vi "Apply.vi"(8 "error in (no error)":errorcluster, 11 "PXIe-5172:Fetch Waveforms CFG in":refnum<class "Voltmeter CFG.lvclass">=refnum) -> (0 "error out":errorcluster, 3 "PXIe-5172:Fetch Waveforms CFG out":refnum<class "Voltmeter CFG.lvclass">)   [LabVIEW 2023, in "PXIe-5172.lvlib" / "Fetch Waveforms CFG.lvclass"]
uses:
  Fetch Waveforms CFG.lvclass
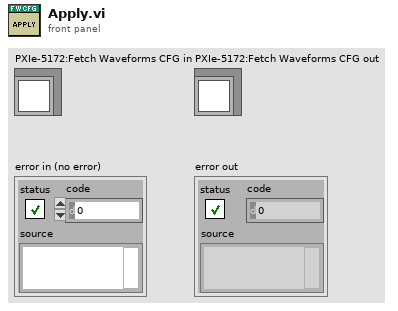
[diagram p1: front panel]
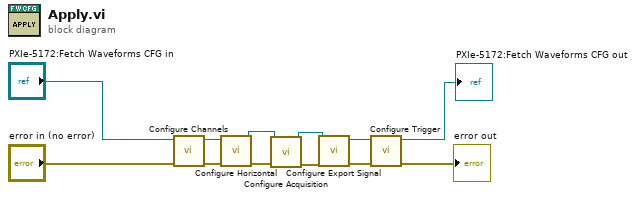
[diagram p0: block diagram]
diagram:
  n1 = call-dynamic "Configure Channels.vi"("error in"="error in (no error)", "Scope PXI CFG in"="PXIe-5172:Fetch Waveforms CFG in") -> ("error out"=w11:errorcluster, "Scope PXI CFG out"=w12:refnum<class "Voltmeter CFG.lvclass">)  [unwired: 8 in]
  n2 = call-dynamic "Configure Horizontal.vi"("error in"=w11, "Scope PXI CFG in"=w12) -> ("error out"=w7:errorcluster, "Scope PXI CFG out"=w8:refnum<class "Voltmeter CFG.lvclass">)  [unwired: 8 in]
  n3 = call-dynamic "Configure Acquisition.vi"("error in"=w7, "Scope PXI CFG in"=w8) -> ("error out"=w5:errorcluster, "Scope PXI CFG out"=w6:refnum<class "Voltmeter CFG.lvclass">)  [unwired: 8 in]
  n4 = call-dynamic "Configure Export Signal.vi"("error in"=w5, "Scope PXI CFG in"=w6) -> ("error out"=w3:errorcluster, "Scope PXI CFG out"=w4:refnum<class "Voltmeter CFG.lvclass">)  [unwired: 8 in]
  n5 = call "Configure Trigger.vi"("error in"=w3, "Scope PXI CFG in"=w4) -> ("error out"=→"error out":errorcluster, "Scope PXI CFG out"=→"PXIe-5172:Fetch Waveforms CFG out":refnum<class "Voltmeter CFG.lvclass">)  [unwired: 8 in]
